vi "SVL Power in Band (1 Ch).vi"(0 "spectrum":cluster{"x0":dbl, "dx":dbl, "magnitude":dbl[]} {"magnitude" format="%.2f"; "dx" format="%.2f"; "x0" format="%.2f"}, 1 "range":cluster{"start":dbl, "stop":dbl}={"start"=-1.0, "stop"=-1.0} {"stop" format="%.2f"; "start" format="%.2f"}, 4 "spectrum info":T1={"channel name"="", "description"="", "x-axis units"=0, "spectral info"={"spectrum type"=enum."Power [Magnitude^2]", "linear/dB"=enum."linear", "window"=0, "window size"=0, "FFT size"=0}, "engineering units"=0, "custom label"="", "dB reference [EU]"=0.0, "peak units"=enum."rms", "weighting filter"=0, "spectral density?"=FALSE, "unit label"="", "spectrum skewed?"=FALSE, "complimentary spectrum units"=enum."none"} {"x-axis units" items=["Time (s)"=0, "Frequency-CB (Hz)"=1, "Frequency-CPB (Hz)"=1248, "Frequency-Arbitrary (Hz)"=2357, "Quefrency (s)"=2, "Revolutions (rev)"=3, "Order"=4, "Speed (RPM)"=11, "Speed (rad/s)"=21, "Index"=65535]; "weighting filter" items=["Linear", "A-weighting", "B-weighting", "C-weighting", "ITU-R 468-4", "Dolby", "CCITT", "C-message", "Wb", "Wc", "Wd", "We", "Wf", "Wh", "Wj", "Wk", "Wm", "AES17 20 kHz lowpass", "AES17 40 kHz lowpass", "AES17 20 kHz highpass", "AES17 40 kHz highpass"]; "dB reference [EU]" format="%.2f"; "engineering units" items=["custom..."=0, "V"=1, "A"=21, "C"=30, "pC"=31, "s"=32, "-"=29, "Pa"=2, "N"=20, "g"=3, "m/s^2"=4, "m/s"=5, "m"=6, "mm/s"=12, "mm"=13, "micron/s"=14, "micron"=15, "in/s^2"=7, "in/s"=8, "in"=9, "mil/s"=10, "mil"=11, "rad/s^2"=16, "rad/s"=17, "rad"=18, "deg/s^2"=26, "deg/s"=27, "deg"=28, "RPM"=22, "cycle/s^2"=23, "Hz"=24, "cycle"=25, "strain"=19]; "spectral info"."window" items=["None "=0, "Hanning"=1, "Hamming"=2, "Blackman-Harris"=3, "Exact Blackman"=4, "Blackman"=5, "Flat Top"=6, "4 Term B-Harris "=7, "7 Term B-Harris"=8, "Low Sidelobe"=9, "Force - Exponential"=10, "Gaussian"=62]}, 5 "error in (no error)":errorcluster) -> (14 "power in band":dbl=nan format="%.2f", 15 "unit label":string, 19 "error out":errorcluster)   [LabVIEW 2017]
doc: "Computes the aggregate power in the <B>range</B>. The SVL Power in Band VI operates on Power, PSD, COP, and FFT [Mag] spectra. You can use this polymorphic VI to analyze a single spectrum or N spectra. The data type you wire to the <B>spectrum</B> input determines the polymorphic instance to use."
uses:
  <vilib>/addons/_NISVFA/_Shared subVIs/Controls/svc_Spectrum Info.ctl
  <vilib>/addons/_NISVFA/_Shared subVIs/Controls/svc_X-Axis Units.ctl
  <vilib>/addons/_NISVFA/_Shared subVIs/Controls/svc_Spectrum Type.ctl
  <vilib>/addons/_NISVFA/_Shared subVIs/Controls/svc_Engineering Units Text Ring.ctl
  <vilib>/addons/_NISVFA/_Shared subVIs/Controls/svc_Weighting Filter Text Ring.ctl
  <vilib>/addons/_NISVFA/_Shared subVIs/Controls/svc_Complimentary Spectrum Units.ctl
  <vilib>/addons/_NISVFA/_Spectrum Processing/SVFA Get Spectrum Subset (1 Ch).vi
  <vilib>/addons/_NISVFA/_Spectrum Processing/SVFA Unit Conversion (1 Ch).vi
  <vilib>/addons/_NISVFA/_Spectrum Processing/subVIs/svfa_Conversion Utility (spectrum info).vi
  <vilib>/addons/_NISVFA/_Spectrum Processing/subVIs/svfa_Peak to RMS to Peak2Peak.vi
  <vilib>/addons/_NISVFA/_Spectrum Processing/subVIs/svfa_Mag to Mag2.vi
  <vilib>/addons/_NISVFA/_Spectrum Processing/subVIs/svfa_Linear to dB.vi
  <vilib>/addons/_NISVFA/_Spectrum Processing/subVIs/svfa_dBrefA to dBrefB.vi
  <vilib>/addons/_NISVFA/_Spectrum Processing/subVIs/svfa_Spectrum to Spectral Density.vi
  <vilib>/addons/_NISVFA/_Shared subVIs/Common/svc_Get Weighting Enum and Labels.vi
  <vilib>/addons/_NISVFA/_Shared subVIs/Common/svc_Unit Label Lexical Class.vi
  <vilib>/addons/_NISVFA/_Shared subVIs/Common/svc_Engineering Units to Unit Label.vi
  <vilib>/addons/_NISVFA/_Shared subVIs/Common/svc_Format Value (DBL).vi
  <vilib>/addons/_NISVFA/_Shared subVIs/Common/svc_Build Unit Label for Frequency Range.vi
  <vilib>/addons/_NISVFA/_Shared subVIs/Common/svc_Convert Frequency to Frequency String.vi
  <vilib>/addons/_NISVFA/_Shared subVIs/Common/svc_Check Frequency Range in Spectrum.vi
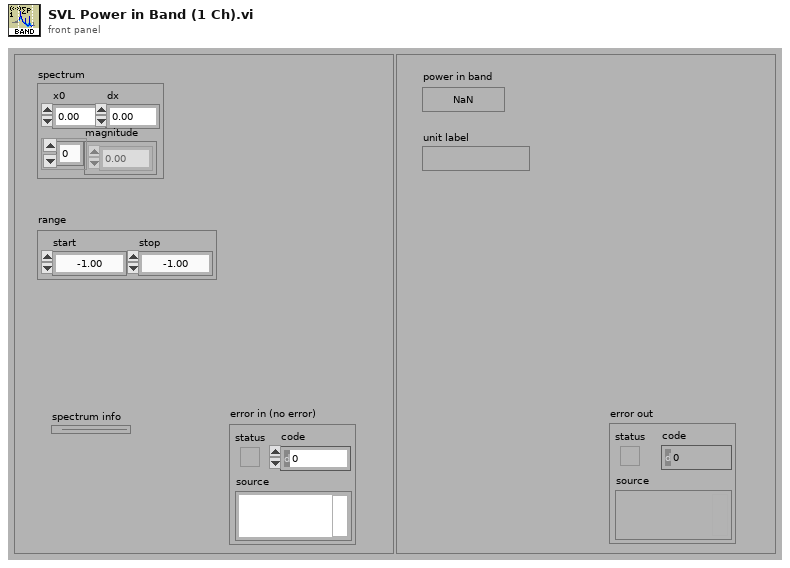
[diagram p1: front panel]
types:
  T1 = typedef "svc_Spectrum Info.ctl" = cluster{"channel name":string, "description":string, "x-axis units":T2, "spectral info":cluster{"spectrum type":T3, "linear/dB":enum16{"linear", "dB"}, "window":u16, "window size":i32, "FFT size":i32}, "engineering units":T4, "custom label":string, "dB reference [EU]":dbl, "peak units":enum16{"rms", "peak", "peak-peak"}, "weighting filter":T5, "spectral density?":bool, "unit label":string, "spectrum skewed?":bool, "complimentary spectrum units":T6}
  T2 = typedef "svc_X-Axis Units.ctl" = u16
  T3 = typedef "svc_Spectrum Type.ctl" = enum16{"FFT Spectrum [complex]", "Amplitude [Magnitude]", "Power [Magnitude^2]", "Cross Spectrum [complex]", "Frequency Response [Complex]"}
  T4 = typedef "svc_Engineering Units Text Ring.ctl" = u16
  T5 = typedef "svc_Weighting Filter Text Ring.ctl" = u16
  T6 = typedef "svc_Complimentary Spectrum Units.ctl" = enum16{"none", "radians", "degrees", "cycles", "imaginary"}
  T7 = cluster{"linear/dB":enum16{"no change", "linear", "dB"}, "dB reference (0: no change)":dbl, "power/magnitude":enum16{"no change", "power", "magnitude"}, "view":enum16{"no change", "rms", "peak", "peak-peak"}}
  T8 = enum16{"no change", "spectrum", "spectral density"}
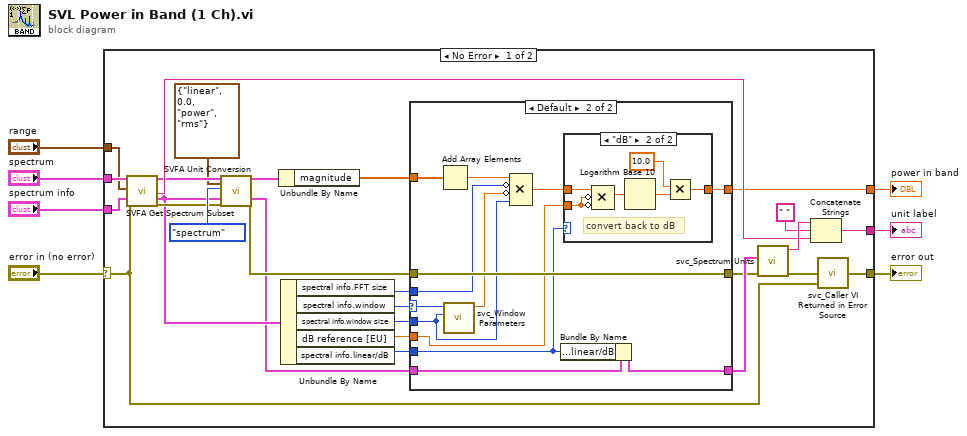
[diagram p0: block diagram]
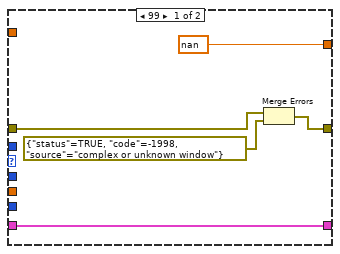
[diagram p2: hidden frame]
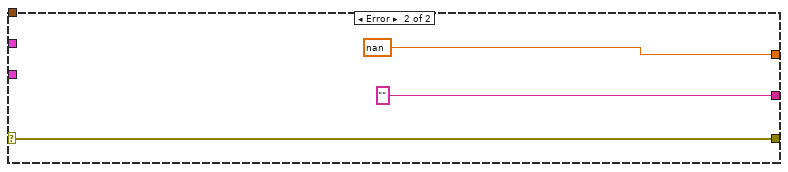
[diagram p4: hidden frame]
diagram:
  n1 = case shown="No Error" "error in (no error)" {
    selector: "error in (no error)" -> [w27 w62]
    tunnel: "spectrum" -> [w26 _]
    tunnel: [w23 nan ("power in band")] -> w6
    tunnel: [w33 w62] -> w5
    tunnel: "range" -> [w22 _]
    tunnel: "spectrum info" -> [w29 _]
    tunnel: [w31 "" ("unit label")] -> w2
    frame No Error {
      n2 = call-poly <vilib>:"SVFA Get Spectrum Subset.vi"("spectrum"=w26, "range"=w22, "spectrum info"=w29, "error in (no error)"=w27) -> ("spectrum subset"=w19:cluster{"x0":dbl, "dx":dbl, "magnitude":dbl[]}, "range label"=w25:string, "dup spectrum info"=w10:T1, "error out"=w15:errorcluster)  [unwired: 10 in, 2 out]
      n3 = call-poly <vilib>:"SVFA Unit Conversion.vi"("spectrum"=w19, "desired scaling"=T7 {"linear/dB"=enum."linear", "dB reference (0: no change)"=0.0, "power/magnitude"=enum."power", "view"=enum."rms"}, "spectral density desired"=T8."spectrum", "spectrum info in"=w10, "error in (no error)"=w15) -> ("converted spectrum"=w18:cluster{"x0":dbl, "dx":dbl, "magnitude":dbl[]}, "spectrum info out"=w9:T1, "error out"=w14:errorcluster)  [unwired: 11 in, 1 out]
      n4 = Unbundle By Name(w18) -> ("magnitude"=w21:dbl[])
      n5 = Unbundle By Name(w10) -> ("spectral info.FFT size"=w12:i32, "spectral info.window"=w20:u16, "spectral info.window size"=w13:i32, "dB reference [EU]"=w8:dbl, "spectral info.linear/dB"=w11:enum16{"linear", "dB"})
      n6 = case shown="Default" w20 {
        selector: w20 -> [_ w47]
        tunnel: [nan w52] -> w23
        tunnel: w21 -> [_ w51]
        tunnel: w14 -> [w39 w50]
        tunnel: [w37 w50] -> w24
        tunnel: w9 -> [w35 w49]
        tunnel: [w35 w48] -> w28
        tunnel: w13 -> [_ w46]
        tunnel: w12 -> [_ w45]
        tunnel: w11 -> [_ w44]
        tunnel: w8 -> [_ w40]
        frame 99 {
          n7 = Merge Errors(w39, errorcluster {"status"=TRUE, "code"=-1998, "source"="complex or unknown window"} ("error out")) -> (w37:errorcluster)
        }
        frame Default {
          n8 = Add Array Elements(numeric array=w51) -> (sum=w42:dbl)
          n9 = call <vilib>:"svc_Window Parameters.vi"("window size"=w46, "window"=w47) -> ("ENBW"=w41:dbl)  [unwired: 6 in, 3 out]
          n10 = Compound Arithmetic op=MULTIPLY(w42, invert w45, invert w41, w46) -> (w43:dbl)
          n11 = Bundle By Name(cluster=w49, "spectral info.linear/dB"=w44) -> (w48:T1)
          n12 = case shown="\"dB\"" w44 {
            tunnel: [w53 w59] -> w52
            tunnel: w43 -> [w53 w55]
            tunnel: w40 -> [_ w56]
            frame "linear", Default {
            }
            frame "dB" {
              # "convert back to dB"
              n13 = Compound Arithmetic op=MULTIPLY(w55, invert w56, invert w56) -> (w54:dbl)
              n14 = Logarithm Base 10(1:w54) -> (0:w58:dbl)
              n15 = Multiply(x=10.0 ("Numeric"), y=w58) -> (x*y=w59:dbl)
            }
          }
        }
      }
      n16 = call <vilib>:"svc_Spectrum Units.vi"("error in (no error)"=w24, "spectrum info in"=w28) -> ("error out"=w34:errorcluster, "unit label"=w32:string)  [unwired: 2 in, 2 out]
      n17 = Concatenate Strings(w32, " " ("string"), w25) -> (w31:string)
      n18 = call <vilib>:"svc_Caller VI Returned in Error Source.vi"("warning input to caller"=w27, "error in (no error)"=w34) -> ("error out"=w33:errorcluster)  [unwired: 3 in]
    }
    frame Error {
    }
  }
  "error out" <- w5
  "power in band" <- w6
  "unit label" <- w2
